vi "GripSmart.vi"(8 "error in":errorcluster, 9 "NoWait":bool, 10 "Grip closed (in)":bool, 11 "Servo":T1) -> (0 "error out":errorcluster, 3 "Grip closed (out)":bool)   [LabVIEW 2017, in "RubikLibraryRT.lvlib"]
doc: "Servo gripper VI. \nThree grippers allowed (Left, Front,Right).\nPositions: opened and closed.\n\n1) Configure PWM frequency, conversion from degrees to duty cycle\n2) Assign PWM B channels to servo/gripper\n3) (Smart) Open PWM B channel\n4) Move servo/gripper, to open or close\n\nReturns the final position, so that state might be maintained. \n\nExecution type: Preallocated clone reentrant execution\nThe addition of the case structure is necessary to keep the correct status (channel). Otherwise the status of the VI does not correlate to the corresponding servo. Each servo (hardware) demands its own VI (software)."
uses:
  ServoEnumControl.ctl
  <vilib>/Utility/error.llb/Error Cluster From Error Code.vi
  <vilib>/myRIO/Common/Instrument Driver Framework/myRIO v1.0/PWM/vis/myRIO v1.0 Write PWM.vi
  Projekt-TestOrientationFSM/RubikLibraryRT.lvlib
  <vilib>/myRIO/Instrument Drivers/Onboard IO/PWM/PWM.lvlib
  RubikLibrary.lvlib
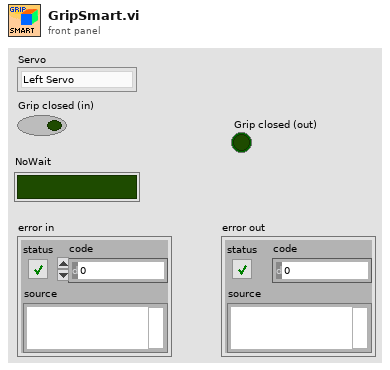
[diagram p1: front panel]
types:
  T1 = typedef "RubikLibrary.lvlib/ServoEnumControl.ctl" = enum16{"Left Servo", "Front Servo", "Right Servo"}
  T2 = typedef "PWM.lvlib/PWM Reference.ctl" = cluster{"myRIO Reference":T3, "PWM Channels Enum":T7, "PWM Configuration":T8}
  T3 = typedef "myRIO Generic Hardware Reference.ctl" = cluster{"myRIO Model":T4, "myRIO Hardware Reference":T5}
  T4 = typedef "Hardware Version Enum.ctl" = enum16{"Unknown", "myRIO-1900", "myRIO-1950", "roboRIO", "NI ELVIS RIO CM"}
  T5 = typedef "myRIO v1.0 Reference.ctl" = cluster{"Generic FPGA Reference":T6, "Allow multiple opens":bool}
  T6 = typedef "Generic FPGA Reference.ctl" = refnum<k20>
  T7 = typedef "PWM Channels Enum.ctl" = enum16{"Not Connected", "C/PWM0", "C/PWM1", "A/PWM0", "A/PWM1", "A/PWM2", "B/PWM0", "B/PWM1", "B/PWM2", "PWM/PWM0", "PWM/PWM1", "PWM/PWM2", "PWM/PWM3", "PWM/PWM4", "PWM/PWM5", "PWM/PWM6", "PWM/PWM7", "PWM/PWM8", "PWM/PWM9"}
  T8 = typedef "PWM.lvlib/PWM Configuration.ctl" = cluster{"Frequency":dbl, "Duty Cycle":dbl}
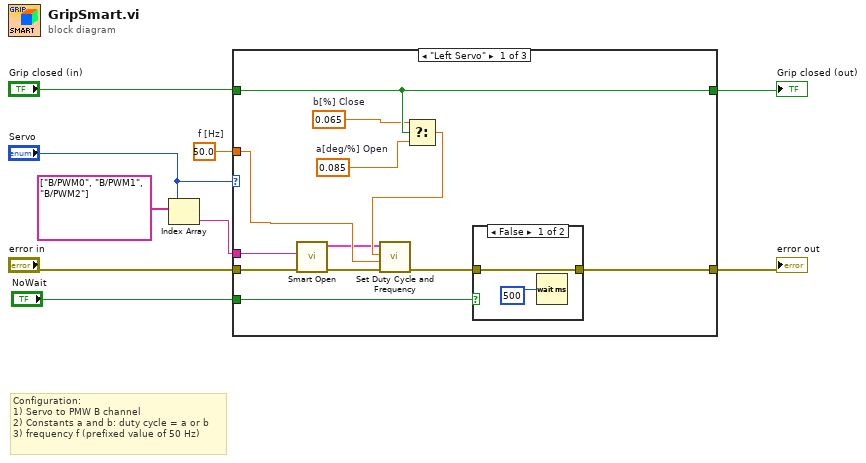
[diagram p0: block diagram]
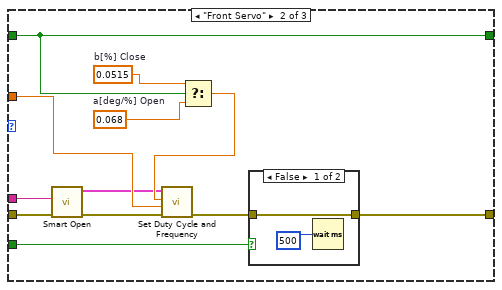
[diagram p3: hidden frame]
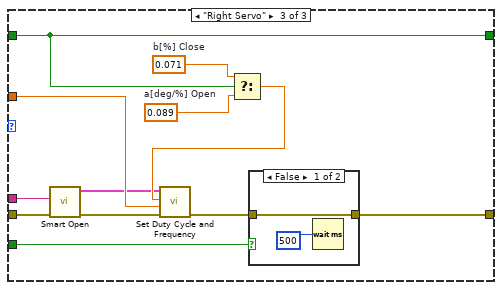
[diagram p5: hidden frame]
diagram:
  w5 = 50.0  # f [Hz]
  # "Configuration:\n1) Servo to PMW B channel\n2) Constants a and b: duty cycle = a or b\n3) frequency f (prefixed value of 50 Hz)"
  n1 = Index Array(array=tag[] ["B/PWM0", "B/PWM1", "B/PWM2"], index="Servo") -> (element=w6:tag)
  n2 = case shown="\"Left Servo\"" "Servo" {
    tunnel: "error in" -> [w19 w36 w49]
    tunnel: [w10 w25 w40] -> w8
    tunnel: w6 -> [w18 w35 w48]
    tunnel: w5 -> [w20 w34 w50]
    tunnel: "Grip closed (in)" -> [w17 w30 w47]
    tunnel: [w17 w30 w47] -> w2
    tunnel: "NoWait" -> [w12 w27 w42]
    frame "Left Servo" {
      w15 = 0.085  # a[deg/%] Open
      w16 = 0.065  # b[%] Close
      n3 = call <vilib>:"Smart Open.vi"("error in (no error)"=w19, "Channel Name"=w18) -> ("error out"=w13:errorcluster, "PWM Ref Out"=w14:T2)  [unwired: 8 in]
      n4 = Select(t=w16, s=w17, f=w15) -> (s? t:f=w21:dbl)
      n5 = call <vilib>:"Set Duty Cycle and Frequency.vi"("error in (no error)"=w13, "Frequency [Hz]"=w20, "Duty Cycle"=w21, "PWM Ref In"=w14) -> ("error out"=w11:errorcluster)  [unwired: 5 in, 1 out]
      n6 = case shown="False" w12 {
        tunnel: w11 -> [w22 w24]
        tunnel: [w22 w24] -> w10
        frame False {
          n7 = Wait (ms)(milliseconds to wait=u32 500) -> ()  [unwired: 1 out]
        }
        frame True {
        }
      }
    }
    frame "Front Servo" {
      w32 = 0.068  # a[deg/%] Open
      w31 = 0.0515  # b[%] Close
      n8 = call <vilib>:"Smart Open.vi"("error in (no error)"=w36, "Channel Name"=w35) -> ("error out"=w28:errorcluster, "PWM Ref Out"=w29:T2)  [unwired: 8 in]
      n9 = Select(t=w31, s=w30, f=w32) -> (s? t:f=w33:dbl)
      n10 = call <vilib>:"Set Duty Cycle and Frequency.vi"("error in (no error)"=w28, "Frequency [Hz]"=w34, "Duty Cycle"=w33, "PWM Ref In"=w29) -> ("error out"=w26:errorcluster)  [unwired: 5 in, 1 out]
      n11 = case shown="False" w27 {
        tunnel: w26 -> [w37 w39]
        tunnel: [w37 w39] -> w25
        frame False {
          n12 = Wait (ms)(milliseconds to wait=u32 500) -> ()  [unwired: 1 out]
        }
        frame True {
        }
      }
    }
    frame "Right Servo" {
      w46 = 0.089  # a[deg/%] Open
      w45 = 0.071  # b[%] Close
      n13 = call <vilib>:"Smart Open.vi"("error in (no error)"=w49, "Channel Name"=w48) -> ("error out"=w43:errorcluster, "PWM Ref Out"=w44:T2)  [unwired: 8 in]
      n14 = Select(t=w45, s=w47, f=w46) -> (s? t:f=w51:dbl)
      n15 = call <vilib>:"Set Duty Cycle and Frequency.vi"("error in (no error)"=w43, "Frequency [Hz]"=w50, "Duty Cycle"=w51, "PWM Ref In"=w44) -> ("error out"=w41:errorcluster)  [unwired: 5 in, 1 out]
      n16 = case shown="False" w42 {
        tunnel: w41 -> [w52 w54]
        tunnel: [w52 w54] -> w40
        frame False {
          n17 = Wait (ms)(milliseconds to wait=u32 500) -> ()  [unwired: 1 out]
        }
        frame True {
        }
      }
    }
  }
  "error out" <- w8
  "Grip closed (out)" <- w2
